vi "evaluateNestedElementWithAttributes.vi"(8 "error in (no error)":errorcluster, 11 "reference in":refnum<class "EasyXML_XML_Subset_Evaluations.lvclass">) -> (0 "error out":errorcluster, 3 "reference in":refnum<class "EasyXML_XML_Subset_Evaluations.lvclass">)   [LabVIEW 2011, in "EasyXML_XML_Subset_Evaluations.lvclass"]
uses:
  EasyXML_XML_Subset_Evaluations.lvclass
panel:
  in  "Entity":T1={"SubEntities"={"Entity"={"#attributes"={"foo"="bar"}}}}
  out "Produced Data":T1
  in  "XML String":string="<Entity>\n  <SubEntities>\n    <Entity foo=\"bar\"/>\n  </SubEntities>\n</Entity>"
  out "Generated XML String":string
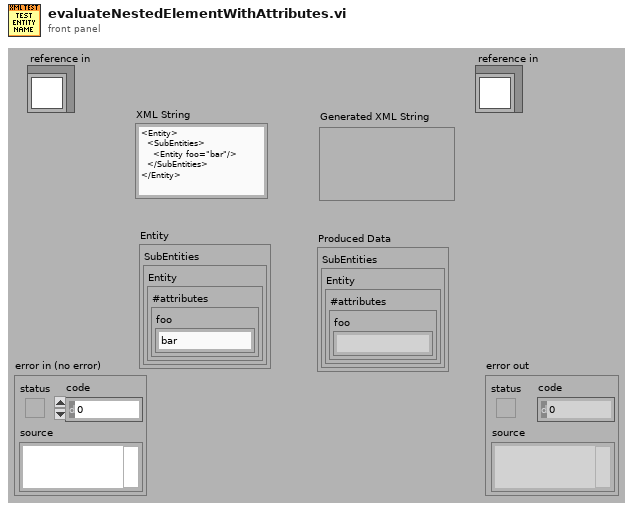
[diagram p1: front panel]
types:
  T1 = cluster{"SubEntities":cluster{"Entity":cluster{"#attributes":cluster{"foo":string}}}}
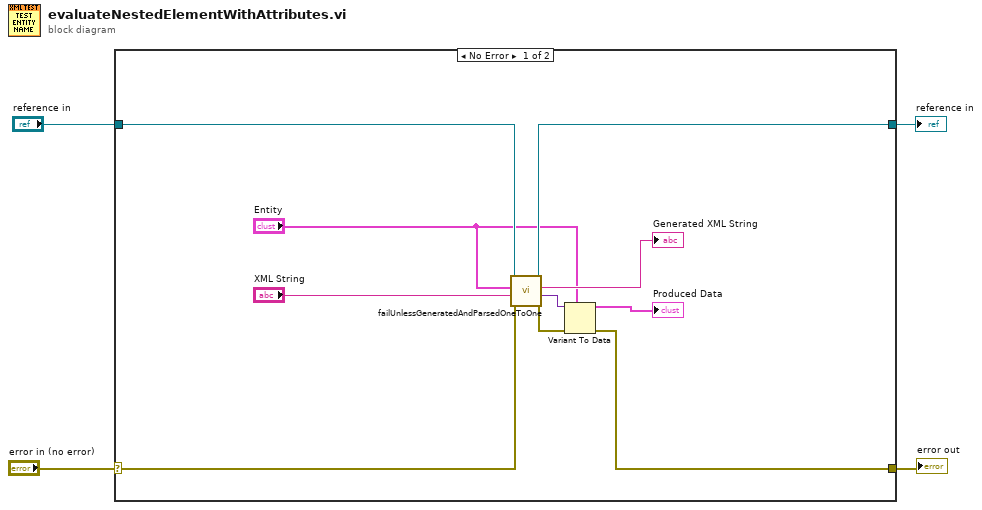
[diagram p0: block diagram]
diagram:
  n1 = case shown="No Error" "error in (no error)" {
    selector: "error in (no error)" -> [w11 w16]
    tunnel: [w5 w16] -> w3
    tunnel: [w13 w15] -> w1
    tunnel: "reference in" -> [w14 w15]
    frame No Error {
      n2 = call "failUnlessGeneratedAndParsedOneToOne.vi"("error in"=w11, "XML String"="XML String", "Data"="Entity", "EasyXMLTest in"=w14) -> ("error out"=w6:errorcluster, "Produced Data"=w9:variant, "Generated XML String"=→"Generated XML String":string, "EasyXMLTest out"=w13:refnum<class "EasyXML_XML_Subset_Evaluations.lvclass">)  [unwired: 4 in]
      n3 = Variant To Data(error in=w6, type="Entity", Variant=w9) -> (data=→"Produced Data":T1, error out=w5:errorcluster)
    }
    frame Error {
    }
  }
  "error out" <- w3
  "reference in" <- w1
